vi "2634КВ022_laser_host.vi"() -> ()   [LabVIEW 2018]
uses:
  Support CTL/Enum_control.ctl
  Support CTL/Tab_typedef.ctl
  <vilib>/Analysis/baseanly.llb/Mean (DBL).vi
  <vilib>/Utility/file.llb/Write Delimited Spreadsheet (string).vi
  <vilib>/Utility/file.llb/Read Delimited Spreadsheet (DBL).vi
  <vilib>/Utility/file.llb/Read From Spreadsheet File (string).vi
  <vilib>/Utility/file.llb/Write To Spreadsheet File (string).vi
  <vilib>/Analysis/NI_AALBase.lvlib
  <vilib>/gmath/NI_Gmath.lvlib
panel:
  out "Путь к точкам":path=path "D:/#mech/LVPROG/1991_Маэстро/Калибровка/Осциллограммы/Точки/0,33"
  in  "Путь к осциллограммам (точки)":path=path "D:/#mech/LVPROG/1991_Маэстро/Калибровка/Осциллограммы/Точки"
  in  "Путь к Офиру":refnum<visa-resource-name>="USB0::0x1AB1::0x04CE::DS1ZB204600526::INSTR"
  in  "Путь к калибровке":path=path "D:/#mech/LVPROG/1991_Маэстро/Калибровка/Дозиметрия офира/1_А_8,88E+6_0,188_1,70E-5_1_25.txt"
  in  "But_Калибровка Ophir":bool
  out "sup_path":path
  out "Имя с интегралом":string
  out "Температура":string
  out "Коэффициент калибровки":string
  out "Отклик":string
  out "Интенсивность 2":string
  out "АРСА/Лазер":string
  out "Номер осциллограммы":string
  in  "Radon":bool
  in  "ОСЦ":bool=TRUE
  out "Точка":dbl=8.0
  in  "Tab Control":T1
  in  "Прострелов в точке":i32
  in  "Текущая точка(2)":i32
  in  "Точки":dbl[](array[numeric])
  in  "Диапазон(F)/Точки(T)":bool
  in  "Текущая точка(1)":i16=1
  in  "Имя файла":string
  out "Интенсивность":dbl
  in  "Конечная интенсивность":dbl
  in  "Начальная интенсивность":dbl
  in  "Количество точек":i16
  out "Интеграл(с учетом П)":dbl
  in  "Гор.Развертка":dbl=0.0001 format="%#_1e"
  in  "Гор.Деление":dbl=5.0 format="%#_1e"
  in  "Верт.Развертка":dbl=1.0 format="%#_1e"
  in  "Верт.Деление":dbl=-3.0 format="%#_1e"
  in  "But_Настройка":bool
  in  "But_Одиночная Фая":bool
  in  "Моща":dbl
  in  "But_Сохранить в CSV":bool
  in  "Название":string
  in  "Курсоры выставлены?":bool
  in  "Перезаписать имя?":bool
  in  "But_Посчитать интеграл":bool
  in  "But_Получить адреса":bool
  out "Интеграл":dbl
  out "Путь осциллограмм":path[](array[path])
  in  "Window Title":string="Select Files:"
  in  "Files of Type 2":string[][](array[string])=[["*.*", "VIs & Controls"], ["*.*", "Sequence Files"], ["*.*", "All Files"]]
  in  "Путь к осциллограммам":path=path "D:/#mech/LVPROG/1991_Маэстро/Калибровка/Осциллограммы"
  out "OSC_address":refnum<visa-resource-name>="USB0::0x1AB1::0x04CE::DS1ZA204619590::INSTR"
  out "Waveform Data":waveform(dbl)(graph)={"t0"=timestamp(0 s since 1904-01-01), "dt"=1e-06, "Y"=array[1200 elements]}
  in  "Путь к осциллографу":refnum<visa-resource-name>="USB0::0x1AB1::0x04CE::DS1ZA204619590::INSTR"
  in  "Channel 2":T2(ring)
  out "Ampermeter_address":refnum<k15>="PXI1Slot4_3 (5)" caption="instrument handle out"
  out "Operation":bool=TRUE
  in  "But_Автопрострел":bool
  in  "Case":T3=enum."Автопрострел"
  in  "But_Получить осциллограмму":bool
  in  "STOP ALL":bool
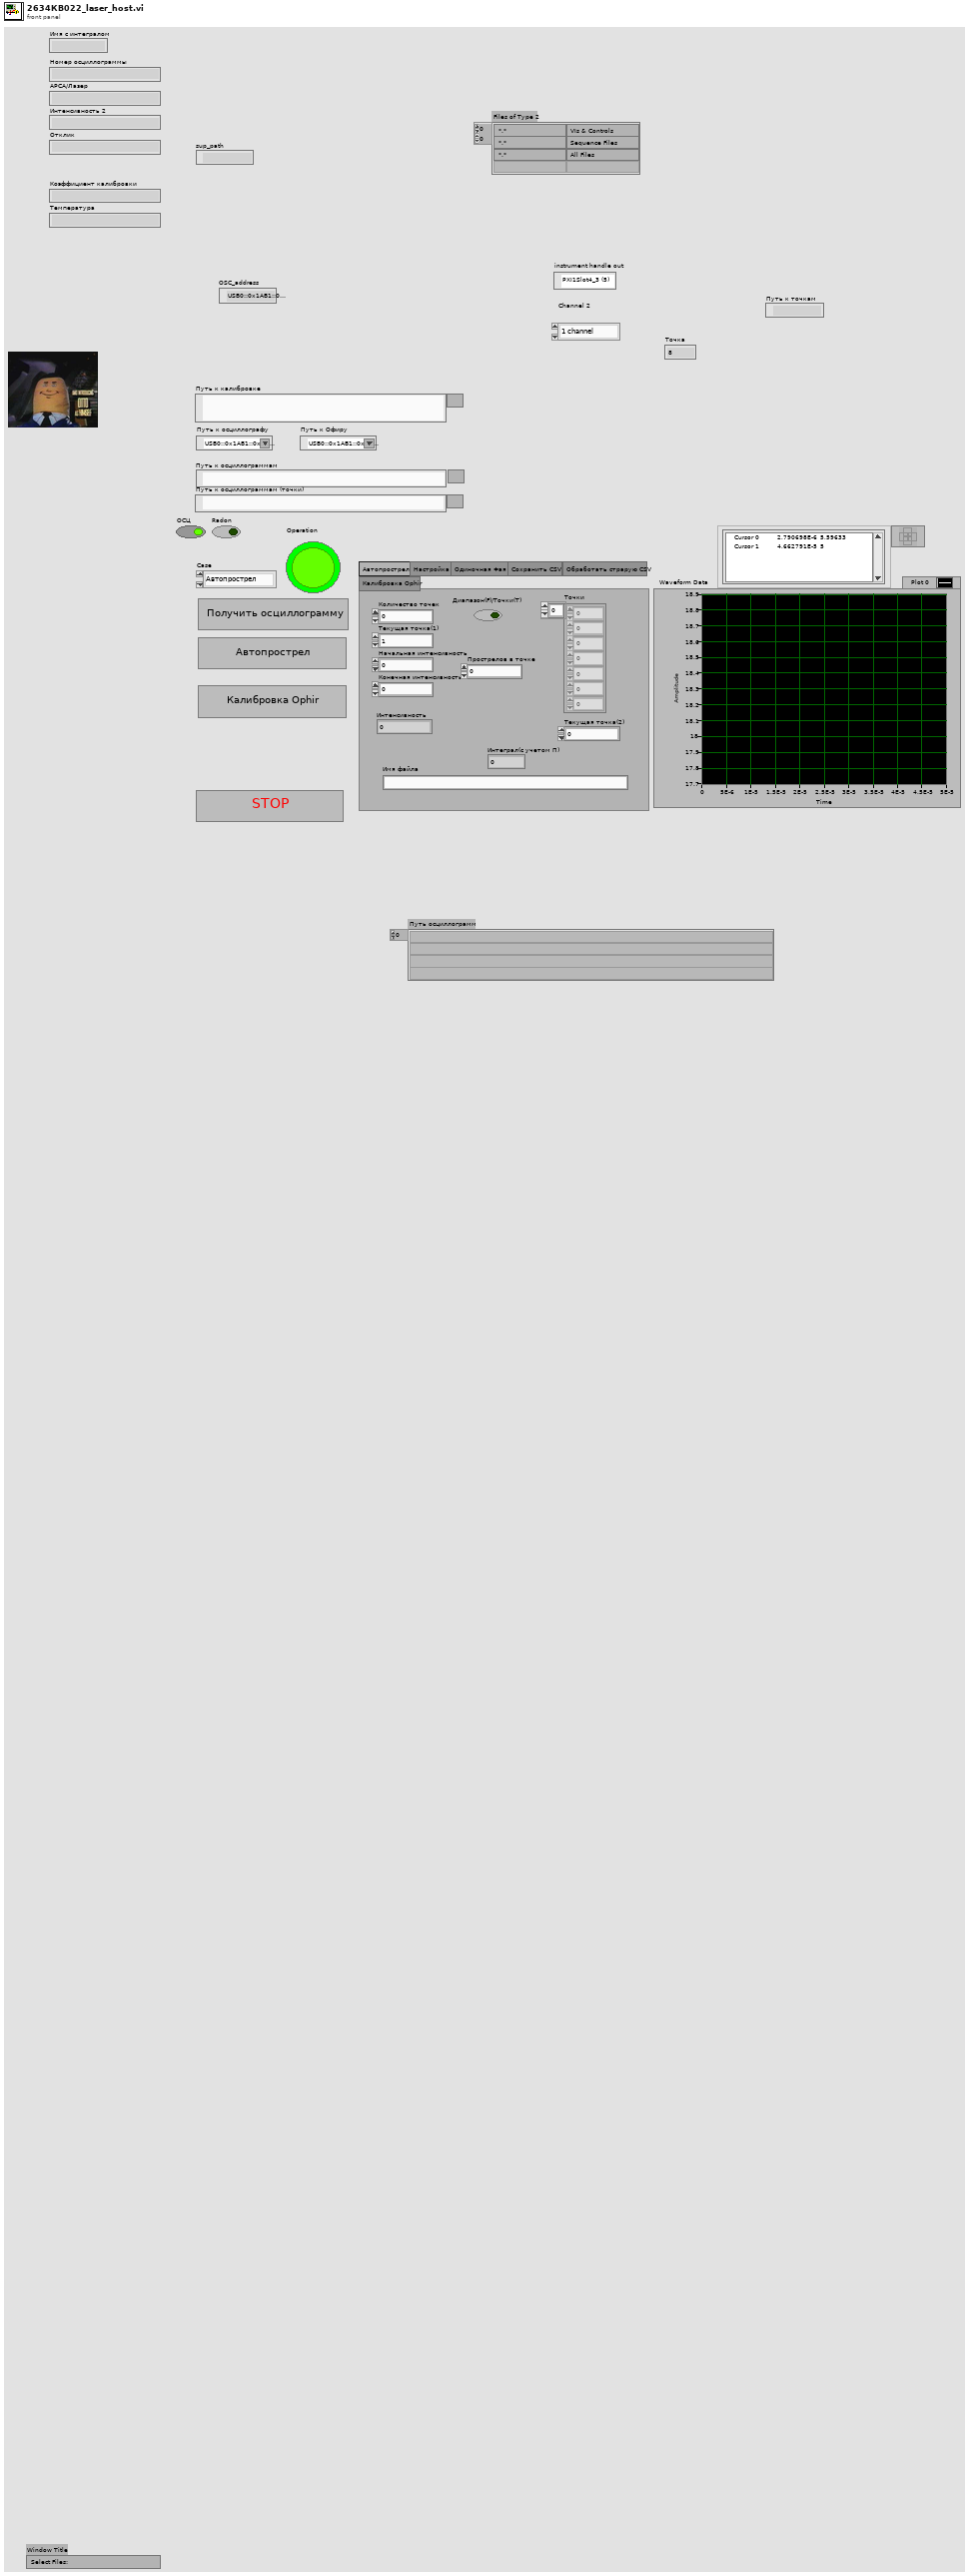
[diagram p1: front panel]
types:
  T1 = typedef "Tab_typedef.ctl" = enum32{"Автопрострел", "Настройка", "Одиночная Фая", "Сохранить CSV", "Обработать страрую CSV", "Калибровка Ophir"}
  T2 = enum16{"1 channel", "2 channel", "3 channel", "4 channel"}
  T3 = typedef "Enum_control.ctl" = enum16{"Калибровка Ophir", "Инициализация", "Посчитать интеграл", "Одиночная Фая", "Ожидание", "Сохранить в CSV", "Автопрострел", "Получить адреса", "Настройка", "Получить осциллограмму"}
  T4 = typedef "LVCursorListTypeDef.ctl" = cluster{"Name":string, "Color":u32, "Style":u8, "Point Style":u8, "Name Visible":bool, "Allow Drag":bool, "Cursor Mode":u32, "Plot":i32, "Index":i32, "Position":cluster{"X":dbl, "Y":dbl}, "X Scale":u32, "Y Scale":u32, "Watch Plots":i32[], "Watch All Plots":bool, "Plot Area":i32, "Label Offset":cluster{"X":dbl, "Y":dbl}}[]
  T5 = cluster{"Name":string, "Color":u32, "Style":u8, "Point Style":u8, "Name Visible":bool, "Allow Drag":bool, "Cursor Mode":u32, "Plot":i32, "Index":i32, "Position":cluster{"X":dbl, "Y":dbl}, "X Scale":u32, "Y Scale":u32, "Watch Plots":i32[], "Watch All Plots":bool, "Plot Area":i32, "Label Offset":cluster{"X":dbl, "Y":dbl}}
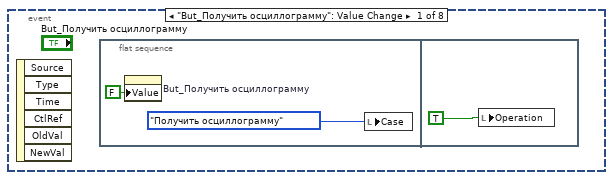
[diagram p2: hidden frame]
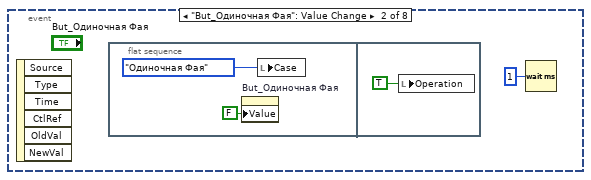
[diagram p3: hidden frame]
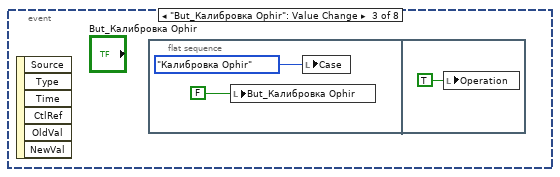
[diagram p4: hidden frame]
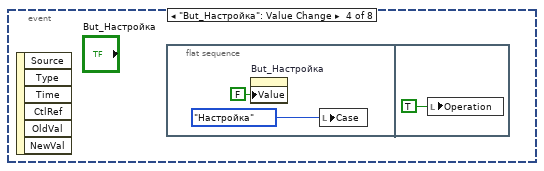
[diagram p5: hidden frame]
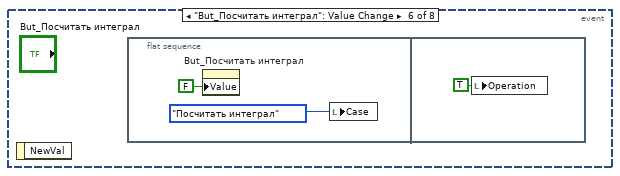
[diagram p6: hidden frame]
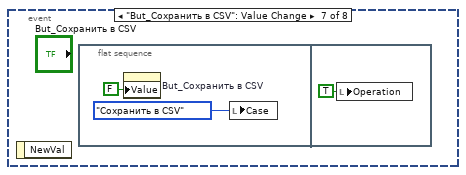
[diagram p7: hidden frame]
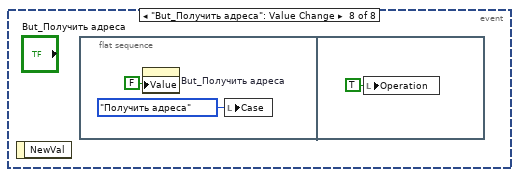
[diagram p8: hidden frame]
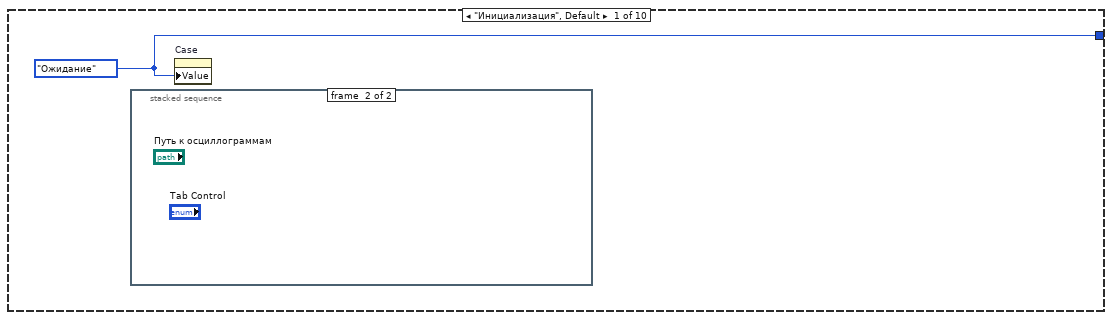
[diagram p9: hidden frame]
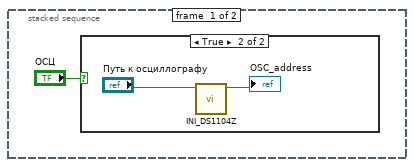
[diagram p10: hidden frame]
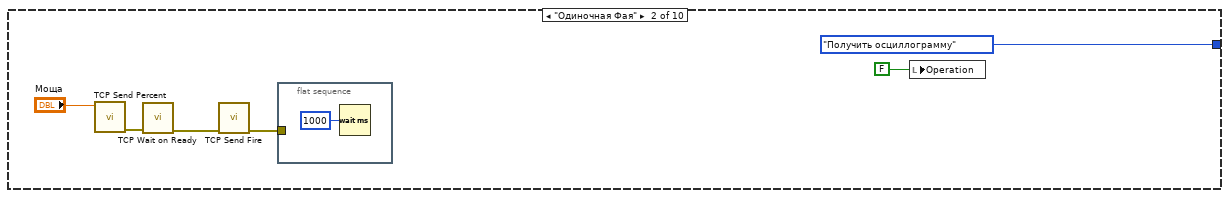
[diagram p12: hidden frame]
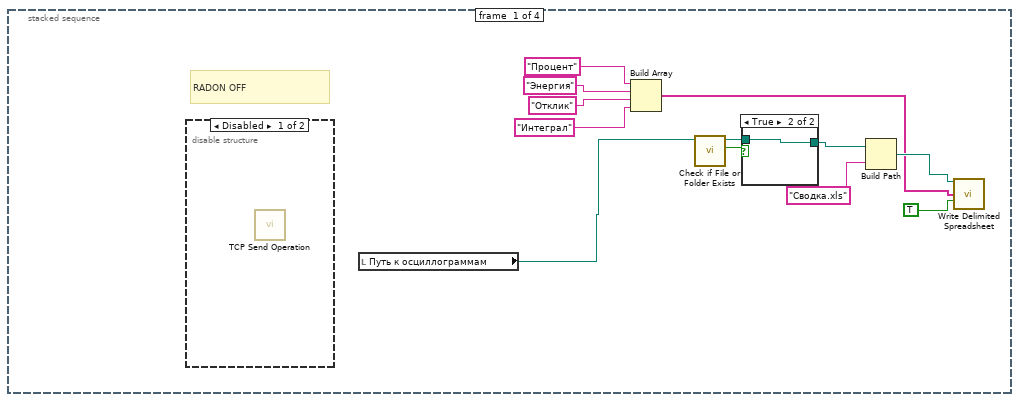
[diagram p13: hidden frame]
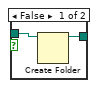
[diagram p15: hidden frame]
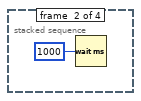
[diagram p16: hidden frame]
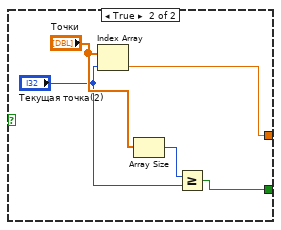
[diagram p17: hidden frame]
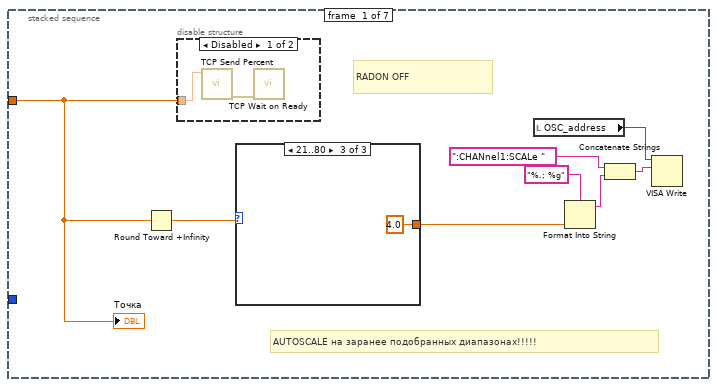
[diagram p18: hidden frame]
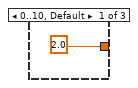
[diagram p20: hidden frame]
diagram:
  (unwired) enum16{"1 channel", "2 channel"}."2 channel" ("Channel")
  (unwired) enum16{"1 channel", "2 channel"}."2 channel" ("Channel")
  (unwired) enum16{"1 channel", "2 channel"}."2 channel" ("Channel")
  (unwired) enum16{"1 channel", "2 channel"}."2 channel" ("Channel")
  # "RADON OFF - 4"
  n1 = flat-sequence {
    tunnel: [w3] -> w1
    frame #0 {
      "Operation" <- FALSE ("Operation")
    }
    frame #1 {
      w3 = Enum_control."Инициализация" ("Case")
      n2 = local write "Case"(w3) -> ()
    }
  }
  n3 = while {
    tunnel: w1 -> [_]
    stop <- FALSE stop-if-true
    n4 = event shown="[4] \"But_Автопрострел\": Value Change" {
      selector: _ -> [_ _ _ _ _ _ _ _]
      dyn-events: _ -> [_ _ _ _ _ _ _ _]
      timeout: _ -> [_ _ _ _ _ _ _ _]
      event "But_Получить осциллограмму": Value Change {
        n5 = event-data() -> ()  [unwired: 1 in, 6 out]
        n6 = flat-sequence {
          frame #0 {
            n7 = property on="But_Получить осциллограмму" class="Bool (strict)"("Value"=FALSE ("But_Read_Data")) -> ()  [unwired: 2 in, 2 out]
            n8 = local write "Case"(Enum_control."Получить осциллограмму" ("Case")) -> ()
          }
          frame #1 {
            n9 = local write "Operation"(TRUE ("Operation")) -> ()
          }
        }
      }
      event "But_Одиночная Фая": Value Change {
        n10 = event-data() -> ()  [unwired: 1 in, 6 out]
        n11 = flat-sequence {
          frame #0 {
            n12 = property on="But_Одиночная Фая" class="Bool (strict)"("Value"=FALSE ("But_Measuring the Output On-Resistancel")) -> ()  [unwired: 2 in, 2 out]
            n13 = local write "Case"(Enum_control."Одиночная Фая" ("Case")) -> ()
          }
          frame #1 {
            n14 = local write "Operation"(TRUE ("Operation")) -> ()
          }
        }
        n15 = Wait (ms)(milliseconds to wait=u32 1) -> ()  [unwired: 1 out]
      }
      event "But_Калибровка Ophir": Value Change {
        n16 = event-data() -> ()  [unwired: 1 in, 6 out]
        n17 = flat-sequence {
          frame #0 {
            n18 = local write "But_Калибровка Ophir"(FALSE ("But_Measuring the Output On-Resistancel")) -> ()
            n19 = local write "Case"(Enum_control."Калибровка Ophir" ("Case")) -> ()
          }
          frame #1 {
            n20 = local write "Operation"(TRUE ("Operation")) -> ()
          }
        }
      }
      event "But_Настройка": Value Change {
        n21 = event-data() -> ()  [unwired: 1 in, 6 out]
        n22 = flat-sequence {
          frame #0 {
            n23 = property on="But_Настройка" class="Bool (strict)"("Value"=FALSE ("But_Write_Data")) -> ()  [unwired: 2 in, 2 out]
            n24 = local write "Case"(Enum_control."Настройка" ("Case")) -> ()
          }
          frame #1 {
            n25 = local write "Operation"(TRUE ("Operation")) -> ()
          }
        }
      }
      event "But_Автопрострел": Value Change {
        n26 = event-data() -> ()  [unwired: 1 in, 1 out]
        n27 = flat-sequence {
          frame #0 {
            n28 = property on="But_Автопрострел" class="Bool (strict)"("Value"=FALSE ("But_Write_Data")) -> ()  [unwired: 2 in, 2 out]
            n29 = local write "Case"(Enum_control."Автопрострел" ("Case")) -> ()
          }
          frame #1 {
            n30 = local write "Operation"(TRUE ("Operation")) -> ()
          }
        }
      }
      event "But_Посчитать интеграл": Value Change {
        n31 = event-data() -> ()  [unwired: 1 in, 1 out]
        n32 = flat-sequence {
          frame #0 {
            n33 = property on="But_Посчитать интеграл" class="Bool (strict)"("Value"=FALSE ("But_Autopilot")) -> ()  [unwired: 2 in, 2 out]
            n34 = local write "Case"(Enum_control."Посчитать интеграл" ("Case")) -> ()
          }
          frame #1 {
            n35 = local write "Operation"(TRUE ("Operation")) -> ()
          }
        }
      }
      event "But_Сохранить в CSV": Value Change {
        n36 = event-data() -> ()  [unwired: 1 in, 1 out]
        n37 = flat-sequence {
          frame #0 {
            n38 = property on="But_Сохранить в CSV" class="Bool (strict)"("Value"=FALSE ("But_Dynamic_read_Current")) -> ()  [unwired: 2 in, 2 out]
            n39 = local write "Case"(Enum_control."Сохранить в CSV" ("Case")) -> ()
          }
          frame #1 {
            n40 = local write "Operation"(TRUE ("Operation")) -> ()
          }
        }
      }
      event "But_Получить адреса": Value Change {
        n41 = event-data() -> ()  [unwired: 1 in, 1 out]
        n42 = flat-sequence {
          frame #0 {
            n43 = property on="But_Получить адреса" class="Bool (strict)"("Value"=FALSE ("But_Dynamic_read_Current")) -> ()  [unwired: 2 in, 2 out]
            n44 = local write "Case"(Enum_control."Получить адреса" ("Case")) -> ()
          }
          frame #1 {
            n45 = local write "Operation"(TRUE ("Operation")) -> ()
          }
        }
      }
    }
  }
  n46 = while {
    shift-right: [w32] -> _
    shift-left: w1 -> [w35]
    stop <- FALSE stop-if-true
    n47 = property on="Operation" class="Bool (strict)"() -> ("Value"=w31:bool)  [unwired: 2 in, 2 out]
    n48 = case shown="True" w31 {
      tunnel: [w522 "Case"] -> w33
      tunnel: w35 -> [w522 _]
      frame False {
      }
      frame True {
      }
    }
    n49 = Wait (ms)(milliseconds to wait=u32 1) -> ()  [unwired: 1 out]
    n50 = case shown="\"Автопрострел\"" w33 {
      tunnel: [w36 Enum_control."Получить осциллограмму" ("Case") w47 Enum_control."Ожидание" ("Case") Enum_control."Ожидание" ("Case") Enum_control."Ожидание" ("Case") Enum_control."Ожидание" ("Case") Enum_control."Ожидание" ("Case") w496 Enum_control."Ожидание" ("Case")] -> w32
      frame "Инициализация", Default {
        w36 = Enum_control."Ожидание" ("Case")
        n51 = stacked-sequence {
          frame #0 {
            n52 = case shown="True" "ОСЦ" {
              frame False {
              }
              frame True {
                n53 = call "INI_DS1104Z.vi"("VISA resource name"="Путь к осциллографу") -> ("VISA resource name out"=→"OSC_address":refnum<visa-resource-name>)  [unwired: 10 in]
              }
            }
          }
          frame #1 {
          }
        }
        n54 = property on="Case" class="Enum (strict)"("Value"=w36) -> ()  [unwired: 2 in, 2 out]
      }
      frame "Одиночная Фая" {
        n55 = call "TCP Send Percent.vi"("Percent"="Моща") -> ("error out"=w41:errorcluster)  [unwired: 10 in]
        n56 = call "TCP Wait on Ready.vi"("error in"=w41) -> ("error out"=w40:errorcluster)  [unwired: 9 in]
        n57 = call "TCP Send Fire.vi"("error in"=w40) -> ("error out"=w42:errorcluster)  [unwired: 10 in]
        n58 = flat-sequence {
          tunnel: w42 -> [_]
          frame #0 {
            n59 = Wait (ms)(milliseconds to wait=u32 1000) -> ()  [unwired: 1 out]
          }
        }
        n60 = local write "Operation"(FALSE ("Operation")) -> ()
      }
      frame "Автопрострел" {
        n61 = stacked-sequence {
          tunnel: [_ _ w64 _] -> w47
          frame #0 {
            # "RADON OFF"
            n62 = disable-structure shown="Disabled" {
              frame Disabled {
                n63 = call "TCP Send Operation.vi"() -> ()  [unwired: 11 in, 1 out]
              }
              frame Enabled {
              }
            }
            n64 = local read "Путь к осциллограммам"() -> (w55:path)
            n65 = Build Array("Процент" ("name or relative path"), "Энергия" ("name or relative path"), "Отклик" ("name or relative path"), "Интеграл" ("name or relative path")) -> (w49:string[])
            n66 = call <vilib>:"Check if File or Folder Exists.vi"("path"=w55) -> ("file or folder exists?"=w59:bool, "dup path"=w58:path)  [unwired: 8 in, 1 out]
            n67 = case shown="True" w59 {
              tunnel: w58 -> [w61 w62]
              tunnel: [w60 w62] -> w57
              frame False {
                n68 = Create Folder(path (use dialog)=w61) -> (created path=w60:path)  [unwired: 2 in, 2 out]
              }
              frame True {
              }
            }
            n69 = Build Path(base path=w57, name or relative path="Сводка.xls") -> (appended path=w50:path)
            n70 = call-poly <vilib>:"Write Delimited Spreadsheet.vi"("file path (dialog if empty)"=w50, "1D data"=w49, "append to file? (new file:F)"=TRUE ("transpose? (no:F)")) -> ()  [unwired: 11 in, 2 out]
          }
          frame #1 {
            n71 = Wait (ms)(milliseconds to wait=u32 1000) -> ()  [unwired: 1 out]
          }
          frame #2 {
            n72 = while {
              tunnel: [w69] -> w64
              stop <- w65 stop-if-true
              n73 = case shown="False" "Диапазон(F)/Точки(T)" {
                tunnel: [w77 w82] -> w70
                tunnel: [w71 w86] -> w67
                frame False {
                  n74 = Subtract(x="Конечная интенсивность", y="Начальная интенсивность") -> (x-y=w80:dbl)
                  n75 = Divide(x=w80, y="Количество точек") -> (x/y=w74:dbl)
                  n76 = Decrement(x="Текущая точка(1)") -> (x-1=w76:i16)
                  n77 = Decrement(x="Текущая точка(1)") -> (x-1=w79:i16)
                  n78 = Greater Or Equal?(x=w79, y="Количество точек") -> (x >= y?=w77:bool)
                  n79 = Multiply(x=w76, y=w74) -> (x*y=w72:dbl)
                  n80 = Add(x=w72, y="Начальная интенсивность") -> (x+y=w71:dbl)
                }
                frame True {
                  n81 = Index Array(array="Точки", index="Текущая точка(2)") -> (element=w86:dbl)
                  n82 = Array Size(array="Точки") -> (size(s)=w84:i32)
                  n83 = Greater Or Equal?(x=w84, y="Текущая точка(2)") -> (x >= y?=w82:bool)
                }
              }
              n84 = case shown="False" w70 {
                tunnel: [w88 Enum_control."Ожидание" ("Case")] -> w69
                tunnel: w67 -> [w90 _]
                tunnel: "Прострелов в точке" -> [w89 _]
                tunnel: [w87 TRUE] -> w65
                frame False {
                  n85 = stacked-sequence {
                    seq-local: [_ _ _ w140 _ _ _] -> [_ _ _ _ w262 w286 _]
                    seq-local: [_ _ _ w139 _ _ _] -> [_ _ _ _ w257 w281 _]
                    tunnel: w90 -> [w93 _ w120 _ w268 w290 _]
                    tunnel: w89 -> [_ _ _ w141 _ _ _]
                    tunnel: [_ _ _ _ _ _ Enum_control."Автопрострел" ("Case")] -> w88
                    tunnel: [_ _ _ _ _ _ FALSE] -> w87
                    frame #0 {
                      # "AUTOSCALE на заранее подобранных диапазонах!!!!!"
                      # "RADON OFF"
                      n86 = Round Toward +Infinity(x=w93) -> (ceil(x): smallest int >= x=w92:dbl)
                      n87 = disable-structure shown="Disabled" {
                        disable-tunnel: w93 -> [w99 _]
                        frame Disabled {
                          n88 = call "TCP Send Percent.vi"("Percent"=w99) -> ("error out"=w100:errorcluster)  [unwired: 10 in]
                          n89 = call "TCP Wait on Ready.vi"("error in"=w100) -> ()  [unwired: 9 in, 1 out]
                        }
                        frame Enabled {
                        }
                      }
                      n90 = case shown="21..80" w92 {
                        tunnel: [2.0 ("Numeric") 3.0 ("Numeric") 4.0 ("Numeric")] -> w91
                        frame 0..10, Default {
                        }
                        frame 11..20 {
                        }
                        frame 21..80 {
                        }
                      }
                      n91 = local read "OSC_address"() -> (w96:refnum<visa-resource-name>)
                      n92 = Format Into String(format string="%.; %g", w91) -> (resulting string=w95:string)  [unwired: 2 in, 1 out]
                      n93 = Concatenate Strings(":CHANnel1:SCALe ", w95) -> (w97:string)
                      n94 = VISA Write(VISA resource name=w96, write buffer=w97) -> ()  [unwired: 1 in, 3 out]
                      "Точка" <- w93
                    }
                    frame #1 {
                      n95 = local read "Путь к калибровке"() -> (w104:path)
                      n96 = local read "Точка"() -> (w110:dbl)
                      n97 = call-poly <vilib>:"Read Delimited Spreadsheet.vi"("file path (dialog if empty)"=w104) -> ("all rows"=w105:dbl[][])  [unwired: 9 in, 5 out]
                      n98 = Initialize Array(w110, 1 ("dimension size")) -> (w109:dbl[])
                      n99 = Index Array(array=w105, index (col)=1 ("disabled index (col)")) -> (element=w113:dbl[])  [unwired: 1 in]
                      n100 = Index Array(array=w105, index (col)=0 ("disabled index (col)")) -> (element=w112:dbl[])  [unwired: 1 in]
                      n101 = call <vilib>:"Interpolate 1D.vi"("xi"=w109, "X"=w112, "Y"=w113) -> ("yi"=w108:dbl[])  [unwired: 6 in, 2 out]
                      n102 = Index Array(array=w108, index=0) -> (element=→"Интенсивность":dbl)
                    }
                    frame #2 {
                      n103 = local read "Имя файла"() -> (w132:string)
                      n104 = Number To Fractional String(number=w120, precision (6)=i16 2) -> (F-format string=w128:string)  [unwired: 2 in]
                      n105 = local read "Интенсивность"() -> (w118:dbl)
                      n106 = Concatenate Strings(w132, w128, "\\" ("string")) -> (w131:string)
                      n107 = local write "Имя файла"(w131) -> ()
                      n108 = Number To Fractional String(number=w118, precision (6)=i16 2) -> (F-format string=w117:string)  [unwired: 2 in]
                      n109 = local read "Путь к осциллограммам (точки)"() -> (w122:path)
                      n110 = call <vilib>:"Check if File or Folder Exists.vi"("path"=w122) -> ("file or folder exists?"=w124:bool, "dup path"=w125:path)  [unwired: 8 in, 1 out]
                      n111 = case shown="False" w124 {
                        tunnel: w125 -> [w134 w135]
                        tunnel: [w133 w135] -> w123
                        frame False {
                          n112 = Create Folder(path (use dialog)=w134) -> (created path=w133:path)  [unwired: 2 in, 2 out]
                        }
                        frame True {
                        }
                      }
                      n113 = Build Path(base path=w123, name or relative path=w117) -> (appended path=w121:path)
                      n114 = call <vilib>:"Check if File or Folder Exists.vi"("path"=w121) -> ("file or folder exists?"=w127:bool, "dup path"=w126:path)  [unwired: 8 in, 1 out]
                      n115 = case shown="False" w127 {
                        tunnel: w126 -> [w137 w138]
                        tunnel: [w136 w138] -> w116
                        frame False {
                          n116 = Create Folder(path (use dialog)=w137) -> (created path=w136:path)  [unwired: 2 in, 2 out]
                        }
                        frame True {
                        }
                      }
                      "Путь к точкам" <- w116
                    }
                    frame #3 {
                      n117 = for {
                        N: w141 -> [_]
                        tunnel: [w143] -> w140 mode=indexing
                        tunnel: [w142] -> w139 mode=indexing
                        i -> [w144]
                        # "Интегралы"
                        # "Амплитуды"
                        n118 = stacked-sequence {
                          tunnel: w144 -> [_ _ _ w151 _ _ _ _ _]
                          tunnel: [_ _ _ _ _ w163 _ _ _] -> w143
                          tunnel: [_ _ _ _ _ _ w196 _ _] -> w142
                          frame #0 {
                            # "RADON OFF"
                            n119 = disable-structure shown="Disabled" {
                              frame Disabled {
                                n120 = call "TCP Send Fire.vi"() -> ()  [unwired: 11 in, 1 out]
                              }
                              frame Enabled {
                              }
                            }
                          }
                          frame #1 {
                            n121 = Wait (ms)(milliseconds to wait=u32 300) -> ()  [unwired: 1 out]
                          }
                          frame #2 {
                            n122 = local read "ОСЦ"() -> (w146:bool)
                            n123 = case shown="True" w146 {
                              frame False {
                              }
                              frame True {
                                w149 = u16 0 items=["Channel 1", "Channel 2", "Channel 3", "Channel 4"] ("Channel (0: Channel 1)")
                                n124 = local read "OSC_address"() -> (w150:refnum<visa-resource-name>)
                                n125 = call "Get_OSC_DS1104Z.vi"("Timeout (10000 ms)"=u32 1000, "Channel (0: Channel 1)"=w149, "VISA resource name"=w150) -> ("Waveform Data"=w147:waveform(dbl))  [unwired: 8 in]
                                n126 = local write "Waveform Data"(w147) -> ()
                              }
                            }
                          }
                          frame #3 {
                            w153 = "_" ("string")
                            n127 = Number To Decimal String(number=w151) -> (decimal integer string=w155:string)  [unwired: 1 in]
                            n128 = Concatenate Strings(w155, w153, "Л" ("string"), w153) -> (w152:string)
                            n129 = local write "Имя файла"(w152) -> ()
                          }
                          frame #4 {
                            n130 = local read "Интенсивность"() -> (w156:dbl)
                            n131 = local read "Имя файла"() -> (w161:string)
                            n132 = Number To Exponential String(number=w156, precision (6)=i16 2) -> (E-format string=w159:string)  [unwired: 2 in]
                            n133 = Concatenate Strings(w161, w159, "_" ("string")) -> (w157:string)
                            n134 = local write "Имя файла"(w157) -> ()
                          }
                          frame #5 {
                            n135 = local read "Waveform Data"() -> (w177:waveform(dbl))
                            n136 = Unbundle By Name(w177) -> ("Y"=w166:dbl[])
                            n137 = Array Size(array=w166) -> (size(s)=w176:i32)
                            n138 = Array Max & Min(array=w166) -> (min index (indices)=w162:i32)  [unwired: 3 out]
                            n139 = Multiply(x=0.015, y=w176) -> (x*y=w173:dbl)
                            n140 = Multiply(x=w176, y=0.985 ("x")) -> (x*y=w172:dbl)
                            n141 = Greater Or Equal?(x=w162, y=w173) -> (x >= y?=w171:bool)
                            n142 = Less Or Equal?(x=w162, y=w172) -> (x <= y?=w170:bool)
                            n143 = And(x=w171, y=w170) -> (x .and. y?=w169:bool)
                            n144 = case shown="True" w169 {
                              tunnel: ["???" ("Имя файла") w180] -> w167
                              tunnel: w166 -> [_ w195]
                              tunnel: w162 -> [_ w192]
                              tunnel: [0.0 w181] -> w163
                              frame False {
                              }
                              frame True {
                                n145 = Decrement(x=w192) -> (x-1=w190:i32)
                                n146 = Increment(x=w192) -> (x+1=w194:i32)
                                n147 = Increment(x=w194) -> (x+1=w193:i32)
                                n148 = Decrement(x=w190) -> (x-1=w191:i32)
                                n149 = Index Array(array=w195, index #1=w194, index #2=w193, index #3=w192, index #4=w191, index #5=w190) -> (element #1=w188:dbl, element #2=w189:dbl, element #3=w187:dbl, element #4=w186:dbl, element #5=w185:dbl)
                                n150 = Compound Arithmetic op=ADD(w188, w189, w187, w186, w185) -> (w184:dbl)
                                n151 = Divide(x=w184, y=5.0) -> (x/y=w181:dbl)
                                n152 = Number To Fractional String(number=w181, precision (6)=i16 3) -> (F-format string=w180:string)  [unwired: 2 in]
                              }
                            }
                            n153 = local read "Имя файла"() -> (w168:string)
                            n154 = Concatenate Strings(w168, w167, "_" ("string")) -> (w164:string)
                            n155 = local write "Имя файла"(w164) -> ()
                          }
                          frame #6 {
                            n156 = property on="Waveform Data" class="WFGraph (strict)"() -> ("CrsrList"=w216:T4)  [unwired: 2 in, 2 out]
                            n157 = local read "Waveform Data"() -> (w217:waveform(dbl))
                            n158 = Index Array(array=w216) -> (element #1=w215:T5, element #2=w214:T5)  [unwired: 2 in]
                            n159 = Unbundle By Name(w215) -> ("Position.X"=w213:dbl)
                            n160 = Unbundle By Name(w214) -> ("Position.X"=w212:dbl)
                            n161 = Unbundle By Name(w217) -> ("Y"=w211:dbl[], "dt"=w197:dbl)
                            n162 = Divide(x=w213, y=w197) -> (x/y=w210:dbl)
                            n163 = Divide(x=w212, y=w197) -> (x/y=w208:dbl)
                            n164 = Split 1D Array(array=w211, index=w210) -> (second subarray=w209:dbl[])  [unwired: 1 out]
                            n165 = Split 1D Array(array=w209, index=w208) -> (first subarray=w207:dbl[])  [unwired: 1 out]
                            n166 = Split 1D Array(array=w207, index=10) -> (first subarray=w199:dbl[], second subarray=w200:dbl[])
                            n167 = call-poly <vilib>:"Mean.vi"("X"=w199) -> ("mean"=w203:dbl)  [unwired: 1 out]
                            n168 = Multiply(x=w203, y=-1.0) -> (x*y=w205:dbl)
                            n169 = Add(x=w205, y=w200) -> (x+y=w202:dbl[])
                            n170 = for {
                              tunnel: w202 -> [w219] mode=indexing
                              shift-right: [w220] -> w198
                              shift-left: 0.0 -> [w218]
                              n171 = Add(x=w219, y=w218) -> (x+y=w220:dbl)
                            }
                            n172 = Multiply(x=w197, y=w198) -> (x*y=w196:dbl)
                            "Интеграл(с учетом П)" <- w196
                          }
                          frame #7 {
                            w226 = "_" ("string")
                            n173 = local read "Интеграл(с учетом П)"() -> (w227:dbl)
                            n174 = local read "Имя файла"() -> (w229:string)
                            n175 = Number To Exponential String(number=w227, precision (6)=i16 2) -> (E-format string=w222:string)  [unwired: 2 in]
                            n176 = Concatenate Strings(w229, w222, w226, "1" ("string"), w226, "25" ("string"), ".csv" ("string")) -> (w223:string)
                            n177 = local write "Имя файла"(w223) -> ()
                          }
                          frame #8 {
                            n178 = local read "Waveform Data"() -> (w237:waveform(dbl))
                            n179 = Unbundle By Name(w237) -> ("Y"=w236:dbl[], "dt"=w235:dbl)
                            n180 = for {
                              tunnel: w236 -> [w243] mode=indexing
                              tunnel: w235 -> [w245]
                              tunnel: [w238] -> w231 mode=indexing
                              i -> [w244]
                              n181 = Multiply(x=w245, y=w244) -> (x*y=w239:dbl)
                              n182 = Number To Fractional String(number=w239, precision (6)=i16 11) -> (F-format string=w240:string)  [unwired: 2 in]
                              n183 = Format Into String(w243) -> (resulting string=w242:string)  [unwired: 3 in, 1 out]
                              n184 = Concatenate Strings(w240, ";" ("string"), w242) -> (w238:string)
                            }
                            n185 = local read "Путь к точкам"() -> (w233:path)
                            n186 = local read "Имя файла"() -> (w232:string)
                            n187 = Build Path(base path=w233, name or relative path=w232) -> (appended path=w234:path)
                            n188 = call-poly <vilib>:"Write Delimited Spreadsheet.vi"("file path (dialog if empty)"=w234, "1D data"=w231, "append to file? (new file:F)"=TRUE) -> ()  [unwired: 11 in, 2 out]
                          }
                        }
                      }
                    }
                    frame #4 {
                      n189 = local read "Интенсивность"() -> (w264:dbl)
                      n190 = Number To Exponential String(number=w264, precision (6)=i16 2) -> (E-format string=w263:string)  [unwired: 2 in]
                      n191 = call-poly <vilib>:"Mean.vi"("X"=w262) -> ("mean"=w260:dbl)  [unwired: 1 out]
                      n192 = call-poly <vilib>:"Mean.vi"("X"=w257) -> ("mean"=w256:dbl)  [unwired: 1 out]
                      n193 = Number To Fractional String(number=w268, precision (6)=i16 2) -> (F-format string=w267:string)  [unwired: 2 in]
                      n194 = local read "Путь к осциллограммам"() -> (w249:path)
                      n195 = Number To Fractional String(number=w260, precision (6)=i16 3) -> (F-format string=w259:string)  [unwired: 2 in]
                      n196 = Number To Exponential String(number=w256, precision (6)=i16 2) -> (E-format string=w255:string)  [unwired: 2 in]
                      n197 = Build Array(w267, w263, w259, w255) -> (w248:string[])
                      n198 = call <vilib>:"Check if File or Folder Exists.vi"("path"=w249) -> ("file or folder exists?"=w254:bool, "dup path"=w253:path)  [unwired: 8 in, 1 out]
                      n199 = case shown="False" w254 {
                        tunnel: w253 -> [w270 w271]
                        tunnel: [w269 w271] -> w252
                        frame False {
                          n200 = Create Folder(path (use dialog)=w270) -> (created path=w269:path)  [unwired: 2 in, 2 out]
                        }
                        frame True {
                        }
                      }
                      n201 = Build Path(base path=w252, name or relative path="Сводка.xls") -> (appended path=w250:path)
                      n202 = call-poly <vilib>:"Write Delimited Spreadsheet.vi"("file path (dialog if empty)"=w250, "1D data"=w248, "append to file? (new file:F)"=TRUE) -> ()  [unwired: 11 in, 2 out]
                    }
                    frame #5 {
                      w282 = "" ("element")
                      n203 = local read "Интенсивность"() -> (w291:dbl)
                      n204 = Number To Exponential String(number=w291, precision (6)=i16 2) -> (E-format string=w288:string)  [unwired: 2 in]
                      n205 = Number To Fractional String(number=w290, precision (6)=i16 2) -> (F-format string=w289:string)  [unwired: 2 in]
                      n206 = Build Array(w289, w288, "" ("element")) -> (w285:string[])
                      n207 = for {
                        tunnel: w286 -> [w305] mode=indexing
                        shift-right: [w302] -> w284
                        shift-left: w285 -> [w303]
                        n208 = Number To Fractional String(number=w305, precision (6)=i16 3) -> (F-format string=w304:string)  [unwired: 2 in]
                        n209 = Insert Into Array(array=w303, new element=w304) -> (w302:string[])  [unwired: 1 in]
                      }
                      n210 = local read "Путь к точкам"() -> (w275:path)
                      n211 = Build Array (concatenate)(w284, "\r\n", w282, w282) -> (w280:string[])
                      n212 = for {
                        shift-right: [w300] -> w273
                        shift-left: w280 -> [w301]
                        tunnel: w281 -> [w298] mode=indexing
                        n213 = Number To Exponential String(number=w298, precision (6)=i16 2) -> (E-format string=w297:string)  [unwired: 2 in]
                        n214 = Insert Into Array(array=w301, new element=w297) -> (w300:string[])  [unwired: 1 in]
                      }
                      n215 = call <vilib>:"Check if File or Folder Exists.vi"("path"=w275) -> ("file or folder exists?"=w279:bool, "dup path"=w278:path)  [unwired: 8 in, 1 out]
                      n216 = case shown="False" w279 {
                        tunnel: w278 -> [w295 w296]
                        tunnel: [w294 w296] -> w277
                        frame False {
                          n217 = Create Folder(path (use dialog)=w295) -> (created path=w294:path)  [unwired: 2 in, 2 out]
                        }
                        frame True {
                        }
                      }
                      n218 = Build Path(base path=w277, name or relative path="Сводка_точки.xls") -> (appended path=w274:path)
                      n219 = call-poly <vilib>:"Write Delimited Spreadsheet.vi"("file path (dialog if empty)"=w274, "1D data"=w273, "append to file? (new file:F)"=TRUE) -> ()  [unwired: 11 in, 2 out]
                    }
                    frame #6 {
                      n220 = local read "Диапазон(F)/Точки(T)"() -> (w309:bool)
                      n221 = case shown="False" w309 {
                        frame False {
                          n222 = local read "Текущая точка(1)"() -> (w310:i16)
                          n223 = Increment(x=w310) -> (x+1=w311:i16)
                          n224 = local write "Текущая точка(1)"(w311) -> ()
                        }
                        frame True {
                          n225 = local read "Текущая точка(2)"() -> (w312:i32)
                          n226 = Increment(x=w312) -> (x+1=w313:i32)
                          n227 = local write "Текущая точка(2)"(w313) -> ()
                        }
                      }
                    }
                  }
                }
                frame True {
                  n228 = local read "Диапазон(F)/Точки(T)"() -> (w315:bool)
                  n229 = case shown="True" w315 {
                    frame False {
                      n230 = local write "Текущая точка(1)"(i16 1 ("Текущая точка")) -> ()
                    }
                    frame True {
                      n231 = local write "Текущая точка(2)"(0 ("Текущая точка(2)")) -> ()
                    }
                  }
                  n232 = local write "Operation"(FALSE ("Operation")) -> ()
                }
              }
            }
          }
          frame #3 {
            # "RADON OFF"
            n233 = disable-structure shown="Disabled" {
              frame Disabled {
                n234 = call "TCP Send Operation.vi"() -> ()  [unwired: 11 in, 1 out]
              }
              frame Enabled {
              }
            }
          }
        }
      }
      frame "Калибровка Ophir" {
        n235 = call "Ophir_calibration.vi"("Адрес Ophir"="Путь к Офиру", "Путь к калибровке"="Путь к калибровке") -> ()  [unwired: 10 in]
      }
      frame "Посчитать интеграл" {
        n236 = local read "Путь осциллограмм"() -> (w324:path[])
        n237 = for {
          tunnel: w324 -> [w326] mode=indexing
          n238 = stacked-sequence {
            tunnel: w326 -> [w350 _ _ w387 w410 _]
            frame #0 {
              n239 = call-poly <vilib>:"Read From Spreadsheet File.vi"("file path (dialog if empty)"=w350) -> ("all rows"=w349:string[][])  [unwired: 6 in, 4 out]
              n240 = Index Array(array=w349, index (col)=0 ("index (row)")) -> (element=w334:string[])  [unwired: 1 in]
              n241 = Index Array(array=w334, index=1) -> (element=w342:string)
              n242 = Index Array(array=w334, index=2) -> (element=w339:string)
              n243 = for {
                tunnel: w334 -> [w354] mode=indexing
                tunnel: [w353] -> w328 mode=indexing
                n244 = Search and Replace String(replace all?=TRUE ("replace all? (F)"), input string=w354, search string="\"") -> (result string=w356:string)  [unwired: 5 in, 3 out]
                n245 = Match Pattern(string=w356, regular expression=";" ("search string/char (-)")) -> (after substring=w352:string)  [unwired: 1 in, 3 out]
                n246 = Fract/Exp String To Number(string=w352) -> (number=w353:dbl)  [unwired: 3 in, 1 out]
              }
              n247 = Search and Replace String(replace all?=TRUE ("replace all? (F)"), input string=w342, search string="\"") -> (result string=w345:string)  [unwired: 5 in, 3 out]
              n248 = Search and Replace String(replace all?=TRUE ("replace all? (F)"), input string=w339, search string="\"") -> (result string=w336:string)  [unwired: 5 in, 3 out]
              n249 = Match Pattern(string=w345, regular expression=";" ("search string/char (-)")) -> (before substring=w333:string)  [unwired: 1 in, 3 out]
              n250 = Match Pattern(string=w336, regular expression=";" ("search string/char (-)")) -> (before substring=w332:string)  [unwired: 1 in, 3 out]
              n251 = Fract/Exp String To Number(string=w333) -> (number=w330:dbl)  [unwired: 3 in, 1 out]
              n252 = Fract/Exp String To Number(string=w332) -> (number=w331:dbl)  [unwired: 3 in, 1 out]
              n253 = Subtract(x=w331, y=w330) -> (x-y=w329:dbl)
              n254 = To Time Stamp(1:0.0 ("number")) -> (0:w347:timestamp)
              n255 = Bundle By Name("Y"=w328, "dt"=w329, "t0"=w347) -> (w327:waveform(dbl))  [unwired: 1 in]
              n256 = local write "Waveform Data"(w327) -> ()
            }
            frame #1 {
              w359 = FALSE ("Курсоры выставлены?")
              n257 = local write "Курсоры выставлены?"(w359) -> ()
              n258 = while {
                tunnel: w359 -> [_]
                stop <- "Курсоры выставлены?" stop-if-true
                n259 = Wait (ms)(milliseconds to wait=u32 100) -> ()  [unwired: 1 out]
              }
            }
            frame #2 {
              n260 = property on="Waveform Data" class="WFGraph (strict)"() -> ("CrsrList"=w382:T4)  [unwired: 2 in, 2 out]
              n261 = local read "Waveform Data"() -> (w383:waveform(dbl))
              n262 = Index Array(array=w382) -> (element #1=w381:T5, element #2=w380:T5)  [unwired: 2 in]
              n263 = Unbundle By Name(w383) -> ("Y"=w377:dbl[], "dt"=w363:dbl)
              n264 = Unbundle By Name(w381) -> ("Position.X"=w379:dbl)
              n265 = Unbundle By Name(w380) -> ("Position.X"=w378:dbl)
              n266 = Divide(x=w379, y=w363) -> (x/y=w376:dbl)
              n267 = Divide(x=w378, y=w363) -> (x/y=w374:dbl)
              n268 = Split 1D Array(array=w377, index=w376) -> (second subarray=w375:dbl[])  [unwired: 1 out]
              n269 = Split 1D Array(array=w375, index=w374) -> (first subarray=w373:dbl[])  [unwired: 1 out]
              n270 = Split 1D Array(array=w373, index=10) -> (first subarray=w369:dbl[], second subarray=w364:dbl[])
              n271 = call-poly <vilib>:"Mean.vi"("X"=w369) -> ("mean"=w367:dbl)  [unwired: 1 out]
              n272 = Multiply(x=w367, y=-1.0) -> (x*y=w365:dbl)
              n273 = Add(x=w365, y=w364) -> (x+y=w368:dbl[])
              n274 = for {
                tunnel: w368 -> [w385] mode=indexing
                shift-right: [w386] -> w370
                shift-left: 0.0 -> [w384]
                n275 = Add(x=w385, y=w384) -> (x+y=w386:dbl)
              }
              n276 = Multiply(x=w363, y=w370) -> (x*y=→"Интеграл":dbl)
            }
            frame #3 {
              n277 = case shown="True" "Перезаписать имя?" {
                tunnel: w387 -> [_ w389]
                frame False {
                }
                frame True {
                  w400 = "_" ("regular expression")
                  w402 = "_" ("regular expression")
                  n278 = Strip Path(path=w389) -> (name=w409:string)  [unwired: 1 out]
                  n279 = Match Pattern(string=w409, regular expression=w402) -> (before substring=w401:string, after substring=w408:string)  [unwired: 1 in, 2 out]
                  "Номер осциллограммы" <- w401
                  n280 = Match Pattern(string=w408, regular expression=w402) -> (before substring=w399:string, after substring=w407:string)  [unwired: 1 in, 2 out]
                  "АРСА/Лазер" <- w399
                  n281 = Match Pattern(string=w407, regular expression=w402) -> (before substring=w398:string, after substring=w406:string)  [unwired: 1 in, 2 out]
                  "Интенсивность 2" <- w398
                  n282 = Match Pattern(string=w406, regular expression=w402) -> (before substring=w397:string, after substring=w405:string)  [unwired: 1 in, 2 out]
                  "Отклик" <- w397
                  n283 = local read "Интеграл"() -> (w392:dbl)
                  n284 = Match Pattern(string=w405, regular expression=w402) -> (after substring=w404:string)  [unwired: 1 in, 3 out]
                  n285 = Match Pattern(string=w404, regular expression=w402) -> (before substring=w396:string, after substring=w403:string)  [unwired: 1 in, 2 out]
                  "Коэффициент калибровки" <- w396
                  n286 = Number To Exponential String(number=w392, precision (6)=i16 2) -> (E-format string=w391:string)  [unwired: 2 in]
                  n287 = Match Pattern(string=w403, regular expression=w402) -> (before substring=w395:string)  [unwired: 1 in, 3 out]
                  "Температура" <- w395
                  n288 = Concatenate Strings(w401, w400, w399, w400, w398, w400, w397, w400, w391, w400, w396, w400, w395, ".CSV" ("string")) -> (→"Имя с интегралом":string)
                }
              }
            }
            frame #4 {
              n289 = local read "Перезаписать имя?"() -> (w411:bool)
              n290 = case shown="True" w411 {
                tunnel: w410 -> [_ w418]
                frame False {
                }
                frame True {
                  n291 = Strip Path(path=w418) -> (stripped path=w417:path)  [unwired: 1 out]
                  n292 = local read "Waveform Data"() -> (w420:waveform(dbl))
                  n293 = Build Path(base path=w417, name or relative path="1") -> (appended path=w413:path)
                  n294 = Unbundle By Name(w420) -> ("Y"=w423:dbl[], "dt"=w424:dbl)
                  n295 = for {
                    tunnel: w423 -> [w432] mode=indexing
                    tunnel: w424 -> [w431]
                    tunnel: [w429] -> w425 mode=indexing
                    i -> [w430]
                    n296 = Multiply(x=w431, y=w430) -> (x*y=w433:dbl)
                    n297 = Number To Fractional String(use system decimal point (T)=TRUE, number=w433, precision (6)=i16 11) -> (F-format string=w434:string)  [unwired: 1 in]
                    n298 = Format Into String(w432) -> (resulting string=w437:string)  [unwired: 3 in, 1 out]
                    n299 = Concatenate Strings(w434, ";" ("string"), w437) -> (w429:string)
                  }
                  n300 = local read "Имя с интегралом"() -> (w419:string)
                  n301 = call <vilib>:"Check if File or Folder Exists.vi"("path"=w413) -> ("file or folder exists?"=w415:bool, "dup path"=w414:path)  [unwired: 8 in, 1 out]
                  n302 = case shown="False" w415 {
                    tunnel: w414 -> [w427 w428]
                    tunnel: [w426 w428] -> w412
                    frame False {
                      n303 = Create Folder(path (use dialog)=w427) -> (created path=w426:path)  [unwired: 2 in, 2 out]
                    }
                    frame True {
                    }
                  }
                  "sup_path" <- w412
                  n304 = Build Path(base path=w412, name or relative path=w419) -> (appended path=w421:path)
                  n305 = call-poly <vilib>:"Write To Spreadsheet File.vi"("transpose? (no:F)"=TRUE, "1D data"=w425, "file path (dialog if empty)"=w421) -> ()  [unwired: 5 in, 1 out]
                }
              }
            }
            frame #5 {
              n306 = local read "Перезаписать имя?"() -> (w439:bool)
              n307 = case shown="True" w439 {
                frame False {
                }
                frame True {
                  n308 = local read "sup_path"() -> (w451:path)
                  n309 = local read "Интеграл"() -> (w449:dbl)
                  n310 = local read "Номер осциллограммы"() -> (w448:string)
                  n311 = local read "Интенсивность 2"() -> (w447:string)
                  n312 = call <vilib>:"Check if File or Folder Exists.vi"("path"=w451) -> ("file or folder exists?"=w453:bool, "dup path"=w452:path)  [unwired: 8 in, 1 out]
                  n313 = local read "Отклик"() -> (w446:string)
                  n314 = case shown="False" w453 {
                    tunnel: w452 -> [w455 w456]
                    tunnel: [w454 w456] -> w443
                    frame False {
                      n315 = Create Folder(path (use dialog)=w455) -> (created path=w454:path)  [unwired: 2 in, 2 out]
                    }
                    frame True {
                    }
                  }
                  n316 = Number To Exponential String(number=w449, precision (6)=i16 2) -> (E-format string=w445:string)  [unwired: 2 in]
                  n317 = Build Path(base path=w443, name or relative path="Сводка.xls") -> (appended path=w441:path)
                  n318 = Build Array(w448, w447, w446, w445) -> (w444:string[])
                  n319 = call-poly <vilib>:"Write To Spreadsheet File.vi"("append to file? (new file:F)"=TRUE ("transpose? (no:F)"), "1D data"=w444, "file path (dialog if empty)"=w441) -> ()  [unwired: 5 in, 1 out]
                }
              }
            }
          }
        }
        n320 = local write "Operation"(FALSE ("Operation")) -> ()
      }
      frame "Ожидание" {
        n321 = Wait (ms)(milliseconds to wait=u32 100) -> ()  [unwired: 1 out]
      }
      frame "Настройка" {
        n322 = stacked-sequence {
          frame #0 {
            n323 = local write "Tab Control"(Tab_typedef."Настройка" ("Tab Control")) -> ()
            n324 = local read "OSC_address"() -> (w463:refnum<visa-resource-name>)
            n325 = Format Into String(format string="%.; %g", "Гор.Развертка") -> (resulting string=w462:string)  [unwired: 2 in, 1 out]
            n326 = Concatenate Strings(":TIMebase:MAIN:SCALe ", w462) -> (w464:string)
            n327 = VISA Write(VISA resource name=w463, write buffer=w464) -> ()  [unwired: 1 in, 3 out]
          }
          frame #1 {
            n328 = local read "Гор.Развертка"() -> (w470:dbl)
            n329 = Multiply(x=w470, y="Гор.Деление") -> (x*y=w468:dbl)
            n330 = local read "OSC_address"() -> (w471:refnum<visa-resource-name>)
            n331 = Format Into String(format string="%.; %g", w468) -> (resulting string=w475:string)  [unwired: 2 in, 1 out]
            n332 = Concatenate Strings(":TIMebase:MAIN:OFFSet ", w475) -> (w472:string)
            n333 = VISA Write(VISA resource name=w471, write buffer=w472) -> ()  [unwired: 1 in, 3 out]
          }
          frame #2 {
            n334 = local read "OSC_address"() -> (w478:refnum<visa-resource-name>)
            n335 = Format Into String(format string="%.; %g", "Верт.Развертка") -> (resulting string=w477:string)  [unwired: 2 in, 1 out]
            n336 = Concatenate Strings(":CHANnel1:SCALe ", w477) -> (w479:string)
            n337 = VISA Write(VISA resource name=w478, write buffer=w479) -> ()  [unwired: 1 in, 3 out]
          }
          frame #3 {
            n338 = local read "Верт.Развертка"() -> (w484:dbl)
            n339 = Multiply(x=w484, y="Верт.Деление") -> (x*y=w482:dbl)
            n340 = local read "OSC_address"() -> (w486:refnum<visa-resource-name>)
            n341 = Format Into String(format string="%.; %g", w482) -> (resulting string=w485:string)  [unwired: 2 in, 1 out]
            n342 = Concatenate Strings(":CHANnel1:OFFSet ", w485) -> (w487:string)
            n343 = VISA Write(VISA resource name=w486, write buffer=w487) -> ()  [unwired: 1 in, 3 out]
          }
        }
        n344 = local write "Operation"(FALSE ("Operation")) -> ()
      }
      frame "Получить осциллограмму" {
        w492 = u16 0 items=["Channel 1", "Channel 2", "Channel 3", "Channel 4"] ("Channel (0: Channel 1)")
        n345 = local read "OSC_address"() -> (w493:refnum<visa-resource-name>)
        n346 = call "Get_OSC_DS1104Z.vi"("Timeout (10000 ms)"=u32 1000, "Channel (0: Channel 1)"=w492, "VISA resource name"=w493) -> ("Waveform Data"=→"Waveform Data":waveform(dbl))  [unwired: 8 in]
        n347 = local write "Operation"(FALSE ("Operation")) -> ()
      }
      frame "Сохранить в CSV" {
        n348 = stacked-sequence {
          tunnel: [_ Enum_control."Ожидание" ("Case")] -> w496
          frame #0 {
            n349 = local read "Waveform Data"() -> (w504:waveform(dbl))
            n350 = Unbundle By Name(w504) -> ("Y"=w503:dbl[], "dt"=w502:dbl)
            n351 = for {
              tunnel: w503 -> [w510] mode=indexing
              tunnel: w502 -> [w512]
              tunnel: [w505] -> w499 mode=indexing
              i -> [w511]
              n352 = Multiply(x=w512, y=w511) -> (x*y=w506:dbl)
              n353 = Number To Fractional String(number=w506, precision (6)=i16 11) -> (F-format string=w507:string)  [unwired: 2 in]
              n354 = Format Into String(w510) -> (resulting string=w509:string)  [unwired: 3 in, 1 out]
              n355 = Concatenate Strings(w507, ";" ("string"), w509) -> (w505:string)
            }
            n356 = local read "Путь к осциллограммам"() -> (w500:path)
            n357 = Build Path(base path=w500, name or relative path="Название") -> (appended path=w501:path)
            n358 = call-poly <vilib>:"Write To Spreadsheet File.vi"("transpose? (no:F)"=TRUE, "1D data"=w499, "file path (dialog if empty)"=w501) -> ()  [unwired: 5 in, 1 out]
          }
          frame #1 {
            n359 = local write "Operation"(FALSE ("Operation")) -> ()
          }
        }
      }
      frame "Получить адреса" {
        n360 = local read "Путь к осциллограммам"() -> (w517:path)
        n361 = call "Multiple File Selection.vi"("Window Title"="Window Title", "Files of Type In"="Files of Type 2", "Start In"=w517) -> ("Path File Names"=→"Путь осциллограмм":path[])  [unwired: 2 out]
        n362 = local write "Operation"(FALSE ("Operation")) -> ()
      }
    }
  }
  n363 = while {
    stop <- FALSE stop-if-true
    n364 = case shown="False" "STOP ALL" {
      frame False {
        n365 = Wait (ms)(milliseconds to wait=u32 20) -> ()  [unwired: 1 out]
      }
      frame True {
        n366 = stacked-sequence {
          frame #0 {
            n367 = local write "Текущая точка(1)"(i16 1 ("Текущая точка")) -> ()
            n368 = property on="STOP ALL" class="Bool (strict)"("Value"=FALSE ("Power Enable")) -> ()  [unwired: 2 in, 2 out]
            n369 = local write "Case"(Enum_control."Инициализация" ("Case")) -> ()
          }
          frame #1 {
            n370 = Stop(stop? (T)=TRUE) -> ()
          }
        }
      }
    }
  }
